vi "getAllChildren.vi"(8 "error in (no error)":errorcluster, 9 "Child Tag in":string, 11 "Tree ref in":refnum<vi>) -> (0 "error out":errorcluster, 1 "Values":string[](array[string]), 2 "Value Type":string, 3 "Tree ref out":refnum<vi>, 5 "All children out":string[](array[string]))   [LabVIEW 2022 SP3, in "Property Editor.lvlib"]
uses:
  <instrlib>/openDAQ/Examples/Property Editor/Property Editor.lvlib
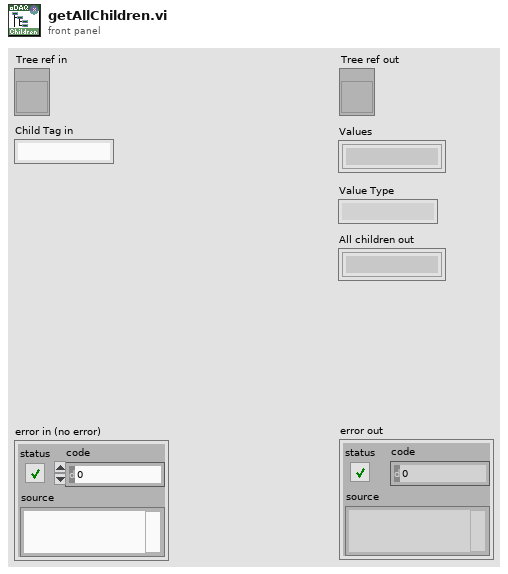
[diagram p1: front panel]
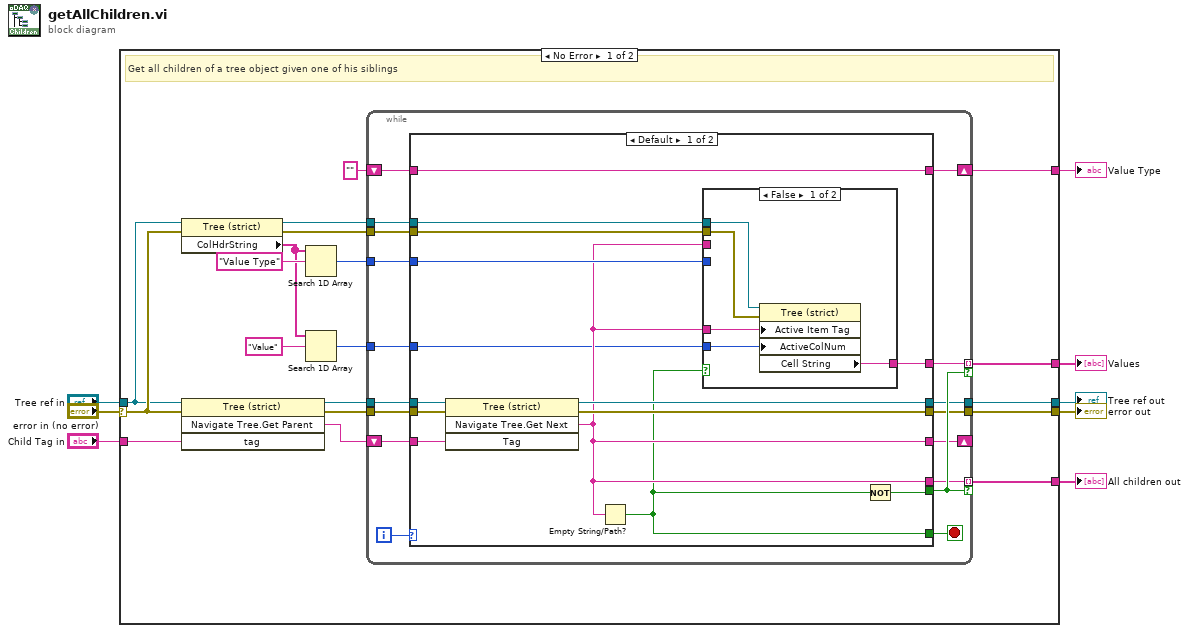
[diagram p0: block diagram]
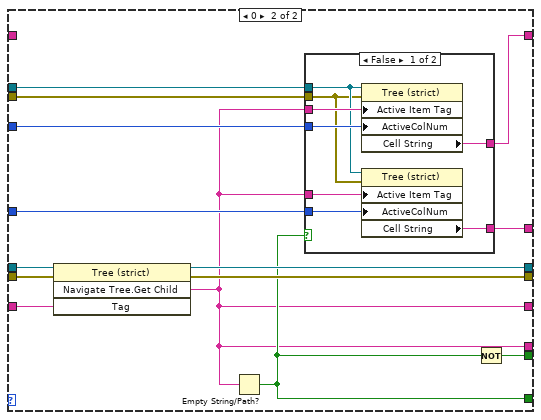
[diagram p3: hidden frame]
diagram:
  n1 = case shown="No Error" "error in (no error)" {
    selector: "error in (no error)" -> [w27 w87]
    tunnel: "Tree ref in" -> [w19 w86]
    tunnel: "Child Tag in" -> [w26 _]
    tunnel: [w22 _] -> w5
    tunnel: [w21 w87] -> w4
    tunnel: [w20 w86] -> w3
    tunnel: [w11 _] -> w2
    tunnel: [w9 _] -> w1
    frame No Error {
      # "Get all children of a tree object given one of his siblings"
      n2 = property class="Tree (strict)"(reference=w19, error in=w27) -> (reference out=w13:refnum<vi>, error out=w12:errorcluster, "ColHdrString"=w16:string[])
      n3 = invoke class="Tree (strict)" method="Navigate Tree.Get Parent"(reference=w19, error in=w27, "tag"=w26) -> (reference out=w25:refnum<vi>, error out=w24:errorcluster, "Navigate Tree:Get Parent"=w23:string)  [unwired: 1 in, 1 out]
      n4 = Search 1D Array(1D array=w16, element="Value Type") -> (index of element=w15:i32)  [unwired: 1 in]
      n5 = Search 1D Array(1D array=w16, element="Value") -> (index of element=w14:i32)  [unwired: 1 in]
      n6 = while {
        tunnel: w25 -> [w42]
        tunnel: w24 -> [w41]
        shift-right: [w39] -> _
        shift-left: w23 -> [w40]
        tunnel: [w38] -> w22 mode=indexing if=w44
        tunnel: [w36] -> w21
        tunnel: [w35] -> w20
        tunnel: w15 -> [w34]
        tunnel: w14 -> [w33]
        tunnel: w13 -> [w32]
        tunnel: w12 -> [w31]
        tunnel: [w30] -> w11 mode=indexing if=w44
        shift-right: [w29] -> w9
        shift-left: "" ("Cell String") -> [w28]
        i -> [w43]
        stop <- w37 stop-if-true
        n7 = case shown="Default" w43 {
          tunnel: w42 -> [w57 w77]
          tunnel: w41 -> [w56 w76]
          tunnel: w40 -> [w55 w75]
          tunnel: [w48 w66] -> w38
          tunnel: [w48 w66] -> w39
          tunnel: [w46 w71] -> w37
          tunnel: [w53 w73] -> w44
          tunnel: [w54 w74] -> w36
          tunnel: [w52 w72] -> w35
          tunnel: w34 -> [w58 w68]
          tunnel: w33 -> [w47 w67]
          tunnel: w32 -> [w50 w70]
          tunnel: w31 -> [w49 w69]
          tunnel: [w51 w65] -> w30
          tunnel: [w45 w64] -> w29
          tunnel: w28 -> [w45 _]
          frame Default {
            n8 = invoke class="Tree (strict)" method="Navigate Tree.Get Next"(reference=w57, error in=w56, "Tag"=w55) -> (reference out=w52:refnum<vi>, error out=w54:errorcluster, "Navigate Tree:Get Next Item"=w48:string)  [unwired: 1 in, 1 out]
            n9 = Empty String/Path?(string/path=w48) -> (empty?=w46:bool)
            n10 = case shown="False" w46 {
              tunnel: w50 -> [w63 _]
              tunnel: w49 -> [w62 _]
              tunnel: w48 -> [_ _]
              tunnel: w58 -> [_ _]
              tunnel: w47 -> [w61 _]
              tunnel: w48 -> [w60 _]
              tunnel: [w59 _] -> w51
              frame False {
                n11 = property class="Tree (strict)"(reference=w63, error in=w62, "Active Item Tag"=w60, "ActiveColNum"=w61) -> ("Cell String"=w59:string)  [unwired: 2 out]
              }
              frame True {
              }
            }
            n12 = Not(x=w46) -> (.not. x?=w53:bool)
          }
          frame 0 {
            n13 = invoke class="Tree (strict)" method="Navigate Tree.Get Child"(reference=w77, error in=w76, "Tag"=w75) -> (reference out=w72:refnum<vi>, error out=w74:errorcluster, "Navigate Tree:Get Child"=w66:string)  [unwired: 1 in, 1 out]
            n14 = Empty String/Path?(string/path=w66) -> (empty?=w71:bool)
            n15 = case shown="False" w71 {
              tunnel: w70 -> [w83 _]
              tunnel: w69 -> [w82 _]
              tunnel: w66 -> [w84 _]
              tunnel: w68 -> [w85 _]
              tunnel: w67 -> [w81 _]
              tunnel: w66 -> [w80 _]
              tunnel: [w79 _] -> w64
              tunnel: [w78 _] -> w65
              frame False {
                n16 = property class="Tree (strict)"(reference=w83, error in=w82, "Active Item Tag"=w84, "ActiveColNum"=w85) -> ("Cell String"=w79:string)  [unwired: 2 out]
                n17 = property class="Tree (strict)"(reference=w83, error in=w82, "Active Item Tag"=w80, "ActiveColNum"=w81) -> ("Cell String"=w78:string)  [unwired: 2 out]
              }
              frame True {
              }
            }
            n18 = Not(x=w71) -> (.not. x?=w73:bool)
          }
        }
      }
    }
    frame Error {
    }
  }
  "All children out" <- w5
  "error out" <- w4
  "Tree ref out" <- w3
  "Values" <- w2
  "Value Type" <- w1
